vi "toVariant.vi"(8 "error in (no error)":errorcluster, 11 "BaseMessage in":refnum<class "BaseMessage.lvclass">) -> (0 "error out":errorcluster, 1 "Variant":variant, 2 "Type":i32, 3 "BaseMessage out":refnum<class "BaseMessage.lvclass">)   [LabVIEW 2013, in "BaseMessage.lvclass"]
doc: "Formats the message to a application specific type integer and a variant.\n\nMessages that are of variant type can be used to send messages to the driver itself. The driver will examine all incoming messages and any variant type messages will be interpreted according to the type integer\n\nThe base implementation of this method returns an empty variant and an error"
uses:
  BaseMessage.lvclass
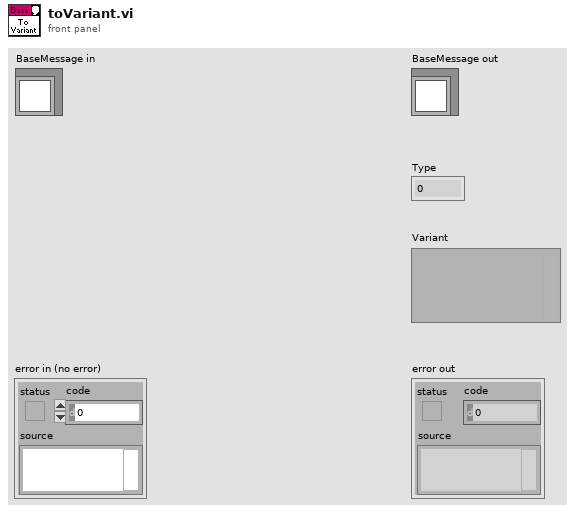
[diagram p1: front panel]
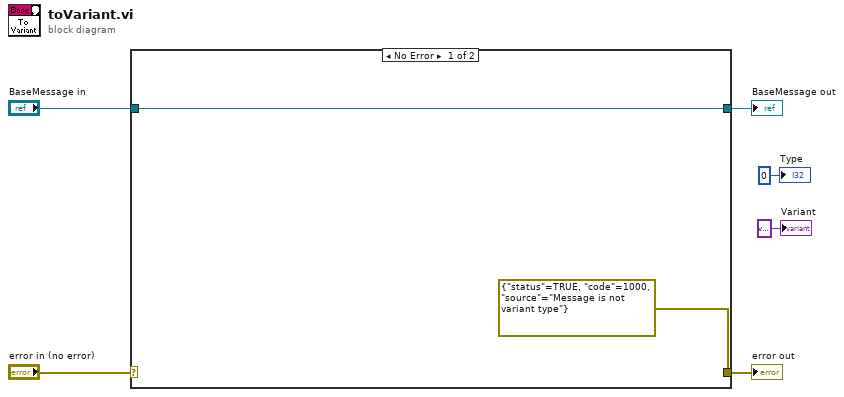
[diagram p0: block diagram]
diagram:
  n1 = case shown="No Error" "error in (no error)" {
    selector: "error in (no error)" -> [_ w10]
    tunnel: [errorcluster {"status"=TRUE, "code"=1000, "source"="Message is not variant type"} ("error IO") w10] -> w5
    tunnel: [w8 w9] -> w3
    tunnel: "BaseMessage in" -> [w8 w9]
    frame No Error {
    }
    frame Error {
    }
  }
  "error out" <- w5
  "BaseMessage out" <- w3
  "Type" <- 0 ("Type")
  "Variant" <- variant ("Variant")
